vi "PM100D_Initialize.vi"() -> (0 "error out":errorcluster, 1 "Instrument":string, 2 "VISA out":refnum<visa-resource-name>, 4 "SN":string)   [LabVIEW 2014]
doc: "This VI scans for connected devices, that can be selected in a dialog box. Next steps\n- setting timeout\n- performing identification query\n- configuring the operation register to '512'; flag gets to HI when a new measurement value is ready to fetch\n- clear operation register"
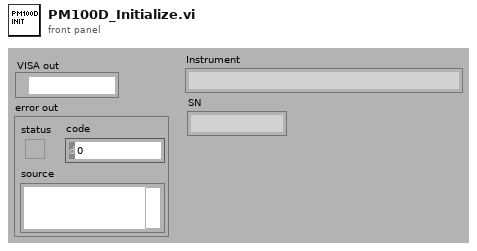
[diagram p1: front panel]
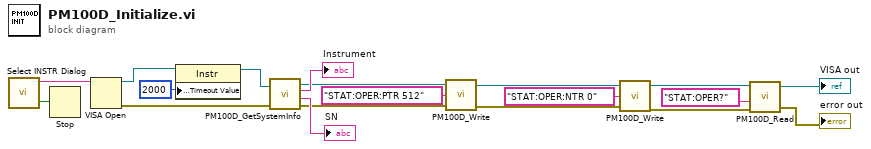
[diagram p0: block diagram]
diagram:
  n1 = call "Select INSTR Dialog.vi"() -> ("Cancel"=w15:bool, "element"=w19:string)  [unwired: 1 in, 2 out]
  n2 = Stop(stop? (T)=w15) -> ()
  n3 = VISA Open(VISA resource name=w19) -> (VISA resource name=w13:refnum<visa-resource-name>, error out=w18:errorcluster)  [unwired: 1 in, 3 out]
  n4 = property class="Instr"(reference=w13, "General Settings:Timeout Value"=u32 2000) -> (reference out=w12:refnum<visa-resource-name>)  [unwired: 1 in, 1 out]
  n5 = call "PM100D_GetSystemInfo.vi"("VISA in"=w12, "error in"=w18) -> ("VISA out"=w10:refnum<visa-resource-name>, "Instrument"=→"Instrument":string, "SN"=→"SN":string, "error out"=w8:errorcluster)
  n6 = call "PM100D_Write.vi"("error in (no error)"=w8, "Command"="STAT:OPER:PTR 512", "VISA in"=w10) -> ("error out"=w7:errorcluster, "VISA out"=w9:refnum<visa-resource-name>)
  n7 = call "PM100D_Write.vi"("error in (no error)"=w7, "Command"="STAT:OPER:NTR 0", "VISA in"=w9) -> ("error out"=w1:errorcluster, "VISA out"=w5:refnum<visa-resource-name>)
  n8 = call "PM100D_Read.vi"("error in (no error)"=w1, "Command"="STAT:OPER?", "VISA in"=w5) -> ("error out"=→"error out":errorcluster, "VISA out"=→"VISA out":refnum<visa-resource-name>)  [unwired: 1 in, 1 out]
